vi "Channel Basics Lesson 5.vi"() -> ()   [LabVIEW 2023]
doc: "This VI demonstrates the ability of channels to go into and out of subVIs and the Call By Reference node."
uses:
  subVIs/Noise Enum.ctl
  <extravilib>/ChannelInstances/Stream-i32/Read With Abort.vi
  <extravilib>/ChannelInstances/Stream-dbl/Read With Abort.vi
  <extravilib>/ChannelInstances/Stream-i32/EndpointRead.vi
  <extravilib>/ChannelInstances/Stream-dbl/EndpointRead.vi
  <extravilib>/ChannelInstances/Stream-dbl/Instantiate.vi
  <extravilib>/ChannelInstances/Stream-dbl/)Channel.vi
  <resource>/ChannelSupport/_ChannelSupport/WaitIfNeeded.vi
  <extravilib>/ChannelInstances/Stream-i32/Instantiate.vi
  <extravilib>/ChannelInstances/Stream-i32/)Channel.vi
  <extravilib>/ChannelInstances/Stream-i32.lvlib
  <extravilib>/ChannelInstances/Stream-dbl.lvlib
panel:
  in  "VI Selection":T1
  out "Reader C":dbl(graph)
  out "Reader B":dbl(graph)
  out "Reader A":i32(graph)
  # "Overview: This VI demonstrates the ability of channels to go into and out of subVIs and the Call By Reference node.\n\nInstructions:\n1. Open the block diagram. Review the lessons presented there.\n2. Select the level of noise to inject into the signal using the VI Selection enum ring.\n3. Run the VI to see the channels in action."
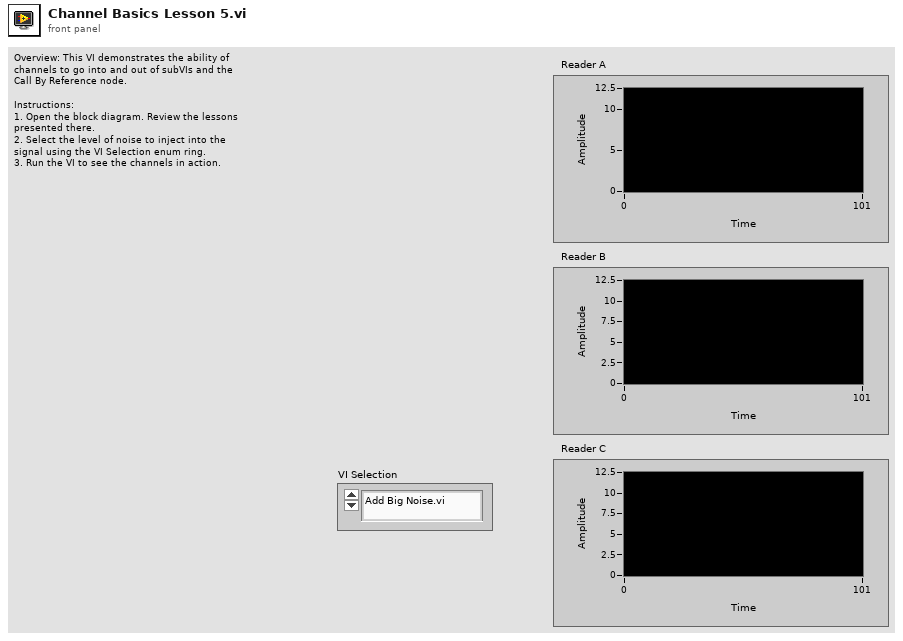
[diagram p1: front panel]
types:
  T1 = typedef "Noise Enum.ctl" = enum16{"Add Big Noise.vi", "Add Small Noise.vi"}
  T2 = typedef "Stream-i32.lvlib/)Channel.ctl" = refnum<queue>
  T3 = typedef "Stream-dbl.lvlib/)Channel.ctl" = refnum<queue>
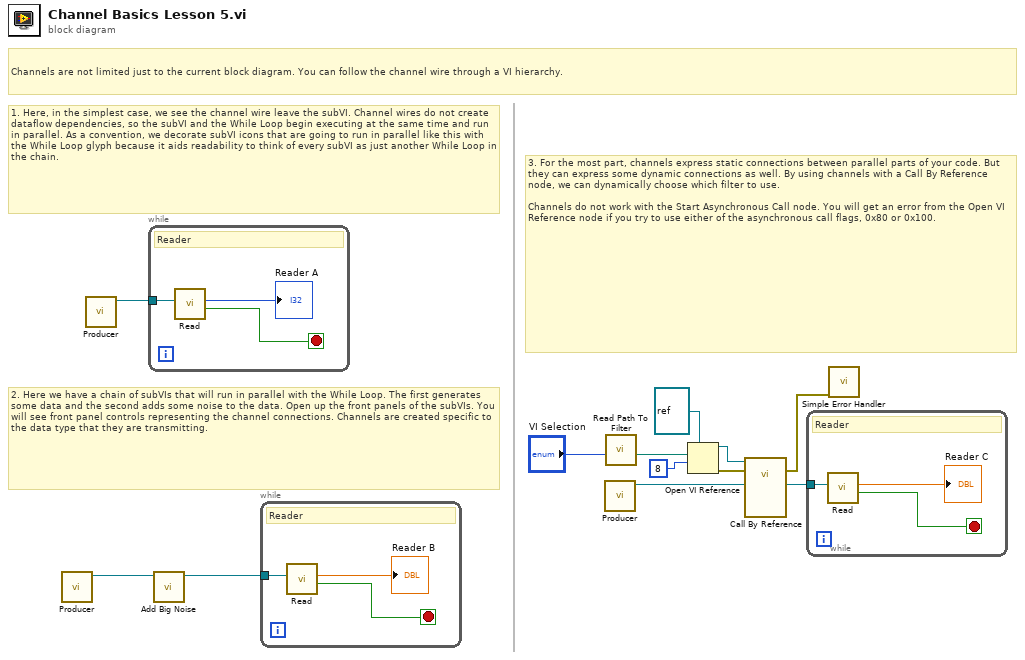
[diagram p0: block diagram]
diagram:
  # "2. Here we have a chain of subVIs that will run in parallel with the While Loop. The first generates some data and the second adds some noise to the data. Open up the front panels of the subVIs. You will see front panel controls representing the channel connections. Channels are created specific to the data type that they are transmitting."
  # "3. For the most part, channels express static connections between parallel parts of your code. But they can express some dynamic connections as well. By using channels with a Call By Reference node, we can dynamically choose which filter to use. \n\nChannels do not work with the Start Asynchronous Call node. You will get an error from the Open VI Reference node if you try to use either of the asynchronous call flags, 0x80 or 0x100."
  # "1. Here, in the simplest case, we see the channel wire leave the subVI. Channel wires do not create dataflow dependencies, so the subVI and the While Loop begin executing at the same time and run in parallel. As a convention, we decorate subVI icons that are going to run in parallel like this with the While Loop glyph because it aids readability to think of every subVI as just another While Loop in the chain."
  # "Channels are not limited just to the current block diagram. You can follow the channel wire through a VI hierarchy."
  n1 = call "Producer.vi"() -> ("channel"=w11:T2)  [unwired: 11 in]
  n2 = call "Producer.vi"() -> ("channel"=w12:T2)  [unwired: 11 in]
  n3 = while {
    tunnel: w12 -> [w15]
    stop <- w13 stop-if-true
    # "Reader"
    n4 = call <extravilib>:"Read.vi"("channel"=w15) -> ("last element?"=w13:bool, "element"=→"Reader A":i32)  [unwired: 6 in, 3 out]
  }
  n5 = call "Add Big Noise.vi"("channel 1"=w11) -> ("channel 2"=w10:T3)  [unwired: 10 in]
  n6 = while {
    tunnel: w10 -> [w18]
    stop <- w16 stop-if-true
    # "Reader"
    n7 = call <extravilib>:"Read.vi"("channel"=w18) -> ("last element?"=w16:bool, "element"=→"Reader B":dbl)  [unwired: 6 in, 3 out]
  }
  n8 = call "Producer.vi"() -> ("channel"=w2:T2)  [unwired: 11 in]
  n9 = call "Read Path To Filter.vi"("VI Name"="VI Selection") -> ("vi path"=w6:path)  [unwired: 10 in]
  n10 = Open VI Reference(type specifier VI Refnum (for type only)=refnum<vi> refnum, vi path=w6, options=8) -> (vi reference=w8:refnum<vi>, error out=w7:errorcluster)  [unwired: 3 in]
  n11 = call-by-ref "?"(reference=w8, error in=w7, "channel 1"=w2) -> (error out=w3:errorcluster, "channel 2"=w1:T3)  [unwired: 10 in, 1 out]
  n12 = while {
    tunnel: w1 -> [w21]
    stop <- w19 stop-if-true
    # "Reader"
    n13 = call <extravilib>:"Read.vi"("channel"=w21) -> ("last element?"=w19:bool, "element"=→"Reader C":dbl)  [unwired: 6 in, 3 out]
  }
  n14 = call <vilib>:"Simple Error Handler.vi"("error in (no error)"=w3) -> ()  [unwired: 4 in, 5 out]
